vi "IIR_SOS_18b_dc_reg.vi"(7 "Coeffs SOS":T1, 8 "enable":bool, 11 "In SOS":fxp<+/-,18,16>) -> (3 "out SOS":fxp<+/-,18,16>)   [LabVIEW 2017]
uses:
  Controls/IIR_Coeffs.ctl
panel:
  out "out":fxp<+/-,24,16>
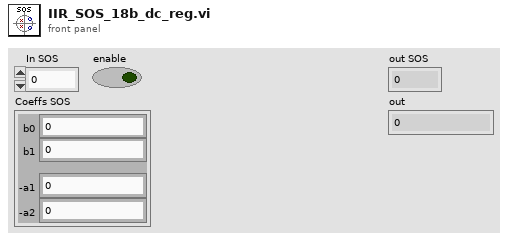
[diagram p1: front panel]
types:
  T1 = typedef "IIR_Coeffs.ctl" = cluster{"b0":fxp<+/-,18,2>, "b1":fxp<+/-,18,2>, "-a1":fxp<+/-,18,2>, "-a2":fxp<+/-,18,2>}
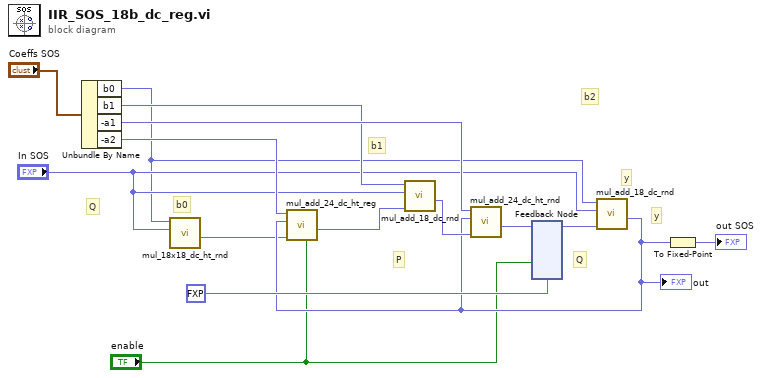
[diagram p0: block diagram]
diagram:
  # "P"
  # "Q"
  # "y"
  # "b1"
  # "b0"
  # "y"
  # "Q"
  # "b2"
  n1 = Unbundle By Name("Coeffs SOS") -> ("b0"=w4:fxp<+/-,18,2>, "b1"=w12:fxp<+/-,18,2>, "-a1"=w14:fxp<+/-,18,2>, "-a2"=w9:fxp<+/-,18,2>)
  n2 = call "mul_18x18_dc_ht_rnd.vi"("Signal"="In SOS", "coeff"=w4) -> ("out"=w3:fxp<+/-,24,16>)  [unwired: 9 in]
  n3 = feedback #1(fxp<+/-,24,16> 0.0) -> (w10:fxp<+/-,24,16>)
  n4 = call "mul_add_18_dc_rnd.vi"("add"=w10, "Signal"="In SOS", "coeff"=w4) -> ("out"=w8:fxp<+/-,24,16>)  [unwired: 8 in]
  "out" <- w8
  n5 = call "mul_add_24_dc_ht_reg.vi"("cep"="enable", "add"=w3, "Signal"=w8, "coeff"=w9) -> ("out"=w2:fxp<+/-,24,16>)  [unwired: 7 in]
  n6 = call "mul_add_18_dc_rnd.vi"("add"=w2, "Signal"="In SOS", "coeff"=w12) -> ("out"=w11:fxp<+/-,24,16>)  [unwired: 8 in]
  n7 = call "mul_add_24_dc_ht_rnd.vi"("add"=w11, "Signal"=w8, "coeff"=w14) -> ("out"=w13:fxp<+/-,24,16>)  [unwired: 8 in]
  n8 = feedback-in #1(w13, "enable") -> ()
  n9 = To Fixed-Point(number=w8) -> (fixed-point=→"out SOS":fxp<+/-,18,16>)  [unwired: 1 in]
